vi "Post-Arm.vi"(8 "error in (no error)":errorcluster, 11 "RP I-V Driver in":refnum<class "RP I-V Driver.lvclass">) -> (0 "error out":errorcluster, 2 "Armed configuration":refnum<class "Start Stream Result.lvclass">, 3 "RP I-V Driver out":refnum<class "RP I-V Driver.lvclass">)   [LabVIEW 2021, in "RP I-V Driver.lvclass"]
uses:
  RP I-V Driver.lvclass
  C:/GitHub/NHMFL_Core/Libraries/Instruments/Pulse Driver/Pulse Driver.lvclass
  Instruments/Results/Start Stream Result/Start Stream Result.lvclass
  Instruments/Pulse Driver/Pulse Driver.lvclass/Pulse Driver.ctl
  Instruments/Pulse Driver/Read t0.vi
  Instruments/Pulse Driver/Write t0.vi
  Red Pitaya Digitizer/Red Pitaya Digitizer.lvclass
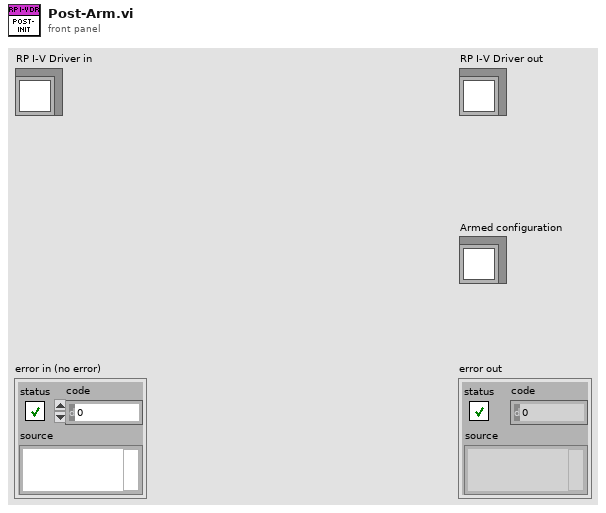
[diagram p1: front panel]
types:
  T1 = typedef "RP I-V Configuration.ctl" = cluster{"I-V parameters":T2, "Ranges":dbl[], "Post-trigger delay":dbl, "Post-trigger duration":dbl, "Output delay":dbl}
  T2 = typedef "I-V parameters.ctl" = cluster{"Start magnitude":dbl, "Magnitude increment":dbl, "End magnitude":dbl, "Ramp length":i32, "Top  length":i32, "Threshold ":dbl, "Processing delay":u16, "Output gain ":dbl, "Interpolation":i32, "Stop after":u16, "Detector window":i32}
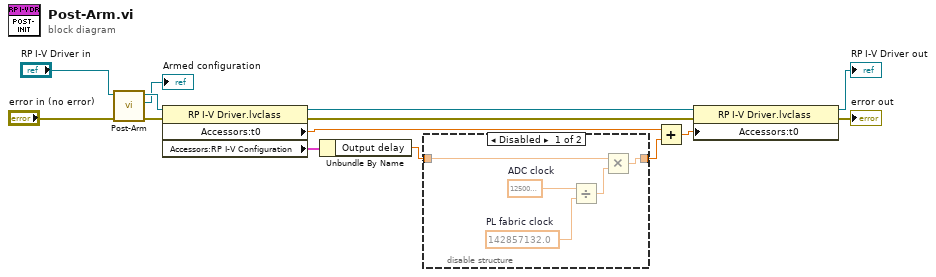
[diagram p0: block diagram]
diagram:
  n1 = call-parent "Post-Arm.vi"("error in (no error)"="error in (no error)", "Pulse Driver in"="RP I-V Driver in") -> ("error out"=w14:errorcluster, "Armed configuration"=→"Armed configuration":refnum<class "Start Stream Result.lvclass">, "Pulse Driver out"=w10:refnum<class "RP I-V Driver.lvclass">)  [unwired: 7 in]
  n2 = property class="RP I-V Driver.lvclass"(reference=w10, error in=w14) -> (reference out=w8:refnum<class "RP I-V Driver.lvclass">, error out=w11:errorcluster, "Accessors:t0"=w5:dbl, "Accessors:RP I-V Configuration"=w6:T1)
  n3 = Unbundle By Name(w6) -> ("Output delay"=w2:dbl)
  n4 = disable-structure shown="Disabled" {
    disable-tunnel: [w17 w20] -> w3
    disable-tunnel: w2 -> [w15 w20]
    frame Disabled {
      w19 = 125000000.0  # ADC clock
      w18 = 142857132.0  # PL fabric clock
      n5 = Divide(x=w19, y=w18) -> (x/y=w16:dbl)
      n6 = Multiply(x=w15, y=w16) -> (x*y=w17:dbl)
    }
    frame Enabled {
    }
  }
  n7 = Add(x=w5, y=w3) -> (x+y=w4:dbl)
  n8 = property class="RP I-V Driver.lvclass"(reference=w8, error in=w11, "Accessors:t0"=w4) -> (reference out=→"RP I-V Driver out":refnum<class "RP I-V Driver.lvclass">, error out=→"error out":errorcluster)
